vi "Dashboard Main.vi"() -> ()   [LabVIEW 2013]
uses:
  Sally_Framework_2014/AutoEnum.ctl
  Sally_Framework_2014/LauncherPresets.ctl
  Sally_Framework_2014/AutoInstructArray.ctl
  Sally_Framework_2014/AutoInstruction.ctl
  <vilib>/event_ctls.llb/eventvkey.ctl
  DBNameEnum.ctl
  <vilib>/Utility/config.llb/Read Key (String).vi
  <vilib>/Utility/config.llb/Read Key (I32).vi
  <vilib>/Utility/config.llb/Write Key (String).vi
  <vilib>/Utility/config.llb/Write Key (I32).vi
  <vilib>/Utility/config.llb/NI_LVConfig.lvlib
panel:
  out "Battery Value":dbl(slide) scale=0.0..14.0 scale format="%#_2e"
  out "Battery":sgl(graph)
  in  "Camera Settings":T1={"Frate Rate"=30, "Compression"=30, "Size"=1} {"Frate Rate" scale=1.0..30.0; "Size" items=["640x480", "320x240", "160x120"]}
  out "Mode":T2(ring)=enum."Auto Disabled"
  out "Camera IP":string
  out "Robot IP":string
  in  "Dashboard Tab":T3(tab)
  out "ReverseDrive":bool
  in  "Use2DriveAlign":bool=TRUE
  out "DriveAlignLSRight":bool
  out "ClimbLS":bool
  in  "UseLauncherPID":bool=TRUE
  in  "UseAngleEncoder":bool=TRUE
  in  "UseLauncherEncoder":bool=TRUE
  out "LauncherAngleMatches":bool
  out "sDriveDistance":dbl
  out "Drive Loop Timing (ms)":u32
  in  "AutoEnum":T4=enum."BehindPyramid"
  out "LauncherMotorValue":dbl
  out "Version":string
  out "LauncherAngle":cluster{dbl, dbl}(knob) scale=0.0..55.0 scale format="%#2_3g"
  out "DriveAlignLSLeft":bool
  out "LauncherRPM":cluster{dbl, dbl}(knob) scale=0.0..4000.0
  in  "Stress TankDrive":bool
  in  "Stress FP":bool
  in  "NumInstr":dbl
  in  "Disabled":T5=[{"Distance/Angle"=10.0, "Speed"=0.0, "Action"=enum."Wait", "NumFrisbees"=0}]
  in  "BehindPyramid":T5=[{"Distance/Angle"=30.0, "Speed"=2390.0, "Action"=enum."Aim", "NumFrisbees"=0}, {"Distance/Angle"=5.0, "Speed"=0.0, "Action"=enum."Wait", "NumFrisbees"=0}, {"Distance/Angle"=0.0, "Speed"=0.0, "Action"=enum."Shoot", "NumFrisbees"=4}]
  in  "CloseLeft":T5=[{"Distance/Angle"=34.0, "Speed"=2390.0, "Action"=enum."Aim", "NumFrisbees"=0}, {"Distance/Angle"=5.0, "Speed"=0.0, "Action"=enum."Wait", "NumFrisbees"=0}, {"Distance/Angle"=0.0, "Speed"=0.0, "Action"=enum."Shoot", "NumFrisbees"=4}]
  in  "CloseRight":T5=[{"Distance/Angle"=34.0, "Speed"=2390.0, "Action"=enum."Aim", "NumFrisbees"=0}, {"Distance/Angle"=5.0, "Speed"=0.0, "Action"=enum."Wait", "NumFrisbees"=0}, {"Distance/Angle"=0.0, "Speed"=0.0, "Action"=enum."Shoot", "NumFrisbees"=4}]
  in  "BackLeft":T5=[{"Distance/Angle"=29.0, "Speed"=2390.0, "Action"=enum."Aim", "NumFrisbees"=0}, {"Distance/Angle"=5.0, "Speed"=0.0, "Action"=enum."Wait", "NumFrisbees"=0}, {"Distance/Angle"=0.0, "Speed"=0.0, "Action"=enum."Shoot", "NumFrisbees"=4}]
  in  "BackRight":T5=[{"Distance/Angle"=29.0, "Speed"=2390.0, "Action"=enum."Aim", "NumFrisbees"=0}, {"Distance/Angle"=5.0, "Speed"=0.0, "Action"=enum."Wait", "NumFrisbees"=0}, {"Distance/Angle"=0.0, "Speed"=0.0, "Action"=enum."Shoot", "NumFrisbees"=4}]
  in  "BackupAuto":dbl[](array[numeric])=[2390.0, 30.0, 3.0, 4.0, 2000.0, -0.5]
  in  "UseClusterArray":bool
  in  "PullbackTol":dbl=100.0
  in  "FireTol":dbl=10.0
  in  "LauncherRPMTol":dbl=10.0
  in  "LauncherAngleTol":dbl=0.1
  in  "InitialWait (ms)":dbl=5000.0
  in  "WaitBetweenLaunch (ms)":dbl=1200.0
  in  "QSWaitBeforeFire (ms)":dbl=600.0
  in  "QSWaitBeforeRetract (ms)":dbl=100.0
  in  "AngleForwardValue":dbl=0.8
  in  "AngleBackwardValue":dbl=-0.8
  in  "HalfSpeedFactor":dbl=0.75
  in  "RPMPresets":T7={"cPresetPyramid"=2390.0, "cPresetShort"=2390.0, "cPresetMid"=1950.0, "cPresetFar"=2390.0, "cPresetClimbHigh"=0.0, "cPresetClimbLow"=0.0}
  in  "AnglePresets":T7={"cPresetPyramid"=30.0, "cPresetShort"=50.0, "cPresetMid"=51.5, "cPresetFar"=25.0, "cPresetClimbHigh"=32.0, "cPresetClimbLow"=20.0}
  in  "Slider":dbl(slide) scale=0.0..100.0 scale format="%#_3g"
  in  "On/Off":bool caption="Solenoid"
  in  "Test Name":u16(ring) items=["Select the test to run...", "Example Test", "-------------------------------", "List of tests is built in robot code.", "Replace with your own automated tests."]
  in  "Test Tree":string(tree)
  in  "Motor":cluster{"Value":dbl, "Enable":bool} {"Value" scale=-1.0..1.0 scale format="%#_3g"}
  out "Progress":T8 {"Test Progress" scale=0.0..100.0}
  in  "Rev/Fwd":cluster{"Forward":bool, "Reverse":bool}
  in  "Ring":u16(ring) items=["Auto", "Fixed indoor", "Fixed outdoor 1", "Fixed outdoor 2", "Fixed fluorescent 1", "Fixed fluorescent 2", "Hold current"]
  in  "Listbox":i32(listbox)=8
  in  "Viewer":T9(tab)
  out "Mbps":dbl format="%#.1g"
  in  "Enable":bool=TRUE
  in  "DB Camera Config":bool
  out "Mbps":bool
  out "fps":dbl format="%#.1g"
  out "Image Error Message":string="Timeout in Camera Communications"
  out "Camera Image":T10(plugin-control)
  out "Buttons 1":cluster{"1":bool, "2":bool, "3":bool}
  out "Kinect 1":cluster{"X":dbl, "Y":dbl, "Z":dbl} {"X" scale=1.0..-1.0; "Y" scale=1.0..-1.0; "Z" scale=1.0..-1.0}
  out "Buttons 2":cluster{"1":bool, "2":bool, "3":bool}
  out "Kinect 2":cluster{"X":dbl, "Y":dbl, "Z":dbl} {"X" scale=1.0..-1.0; "Y" scale=1.0..-1.0; "Z" scale=1.0..-1.0}
  out "Version":string
  out "Skeleton Picture":picture
  out "Players":i8
  out "Tree":string(tree)
  # "Drive & Motors"
  # "Robot IP:"
  # "sLauncherRPM"
  # "TargetLauncherRPM"
  # "sLauncherAngle"
  # "LauncherTargetAngle"
  # "RPM"
  # "Angle"
  # "Wait (s)"
  # "ShootNum"
  # "Time (ms)"
  # "Motor Value"
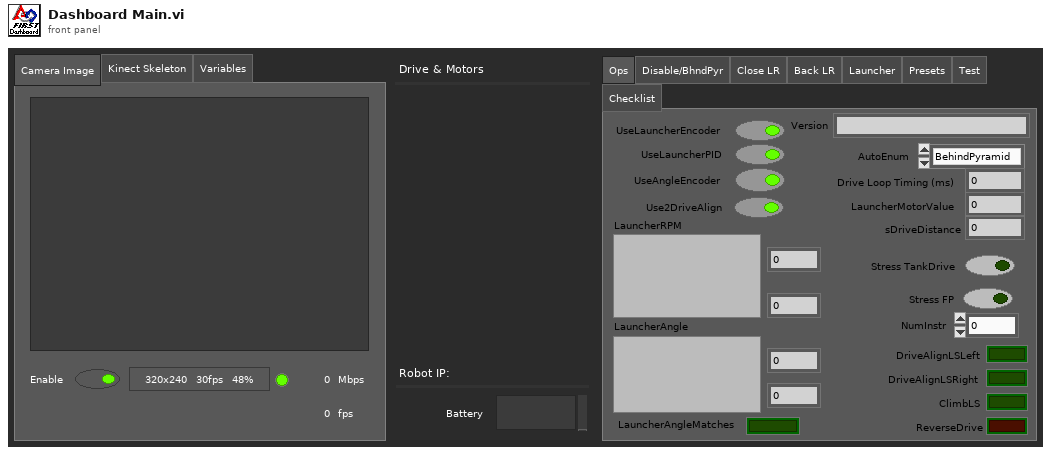
[diagram p1: front panel]
types:
  T1 = cluster{"Frate Rate":i32, "Compression":i32, "Size":u16}
  T2 = enum8{"Tele-Op Disabled", "Tele-Op Enabled", "Auto Disabled", "Auto Enabled", "Test Disabled", "Test Enabled", ""}
  T3 = enum32{"Ops", "Disable/BhndPyr", "Close LR", "Back LR", "Launcher", "Presets", "Test", "Checklist"}
  T4 = typedef "AutoEnum.ctl" = enum16{"Disabled", "BackRight", "BackLeft", "CloseRight", "CloseLeft", "BehindPyramid"}
  T5 = typedef "AutoInstructArray.ctl" = T6[]
  T6 = typedef "AutoInstruction.ctl" = cluster{"Distance/Angle":dbl, "Speed":dbl, "Action":enum16{"DriveForward", "Turn", "Aim", "Shoot", "Wait"}, "NumFrisbees":i32}
  T7 = typedef "LauncherPresets.ctl" = cluster{"cPresetPyramid":dbl, "cPresetShort":dbl, "cPresetMid":dbl, "cPresetFar":dbl, "cPresetClimbHigh":dbl, "cPresetClimbLow":dbl}
  T8 = cluster{"Test Progress":u8, "Test Progress Text":string}
  T9 = enum32{"Camera Image", "Kinect Skeleton", "Variables"}
  T10 = typedef "IMAQ Image.ctl" = refnum<image>
  T11 = typedef "Image Type" = u32
  T12 = typedef "LVBoundsTypeDef.ctl" = cluster{"Width":u32, "Height":u32}
  T13 = typedef "SkeletonTrackState.ctl" = enum32{"NotTracked", "PositionOnly", "Tracked"}
  T14 = cluster{"TrackingState":u8[], "Position":cluster{"x":sgl, "y":sgl, "z":sgl}, cluster{"x":sgl, "y":sgl, "z":sgl, sgl}[], "TrackState":T13}
  T15 = cluster{cluster{"ScaledToPercentRange":dbl, "ScaledToPercentRange":dbl, "ScaledToPercentRange":dbl}, cluster{bool, bool, bool}}[]
  T16 = cluster{cluster{"ScaledToPercentRange":dbl, "ScaledToPercentRange":dbl, "ScaledToPercentRange":dbl}, cluster{bool, bool, bool}}
  T17 = cluster{"ScaledToPercentRange":dbl, "ScaledToPercentRange":dbl, "ScaledToPercentRange":dbl}
  T18 = typedef "LVRectTypeDef.ctl" = cluster{"Left":i16, "Top":i16, "Right":i16, "Bottom":i16}
  T19 = typedef "DBNameEnum.ctl" = enum16{"AutoInstructions", "DriveLoopTime", "DriveAlignLSLeft", "DriveAlignLSRight", "Use2DriveAlign", "ClimbLS", "LauncherAngleMatches", "FrameworkVersion", "sLauncherAngle", "LauncherTargetAngle", "sLauncherRPM", "LauncherTargetRPM", "sDriveDistance", "LauncherMotorValue", "PullbackTol", "FireTol", "LauncherRPMTol", "LauncherAngleTol", "InitialWait", "WaitBetweenLaunch", "AnglePresets", "RPMPresets", "UseAngleEncoder", "UseLauncherEncoder", "UseLauncherPID", "QSWaitBeforeFire", "QSWaitBeforeRetract", "AngleForwardValue", "AngleBackwardValue", "UseClusterArray", "BackupAuto", "ReverseDriveIndicate", "HalfSpeedFactor"}
  T20 = cluster{"Competition mode":bool, "Robot Link":bool, "Autonomous":bool, "Enabled":bool, "E-Stop":bool, "Simulated":bool, "TestMode":bool, "Docked Window":bool}
  T21 = typedef "NI_LVConfig.lvlib/Config Data RefNum.ctl" = refnum<k1>
  T22 = typedef "eventvkey.ctl" = enum16{"ASCII", "Enter", "Return", "Shift", "Ctrl", "Alt", "Cmd", "Opt", "Caps", "NumLock", "Clear", "Break", "Up", "Down", "Left", "Right", "Insert", "Delete", "Home", "End", "PageUp", "PageDown", "Escape", "Help", "Pause", "ScrollLock", "F1", "F2", "F3", "F4", "F5", "F6", "F7", "F8", "F9", "F10", "F11", "F12", "F13", "F14", "F15", "F16", "F17", "F18", "F19", "F20", "F21", "F22", "F23", "F24", "Play", "VolumeUp", "VolumeDown", "Mute", "Two Byte Char"}
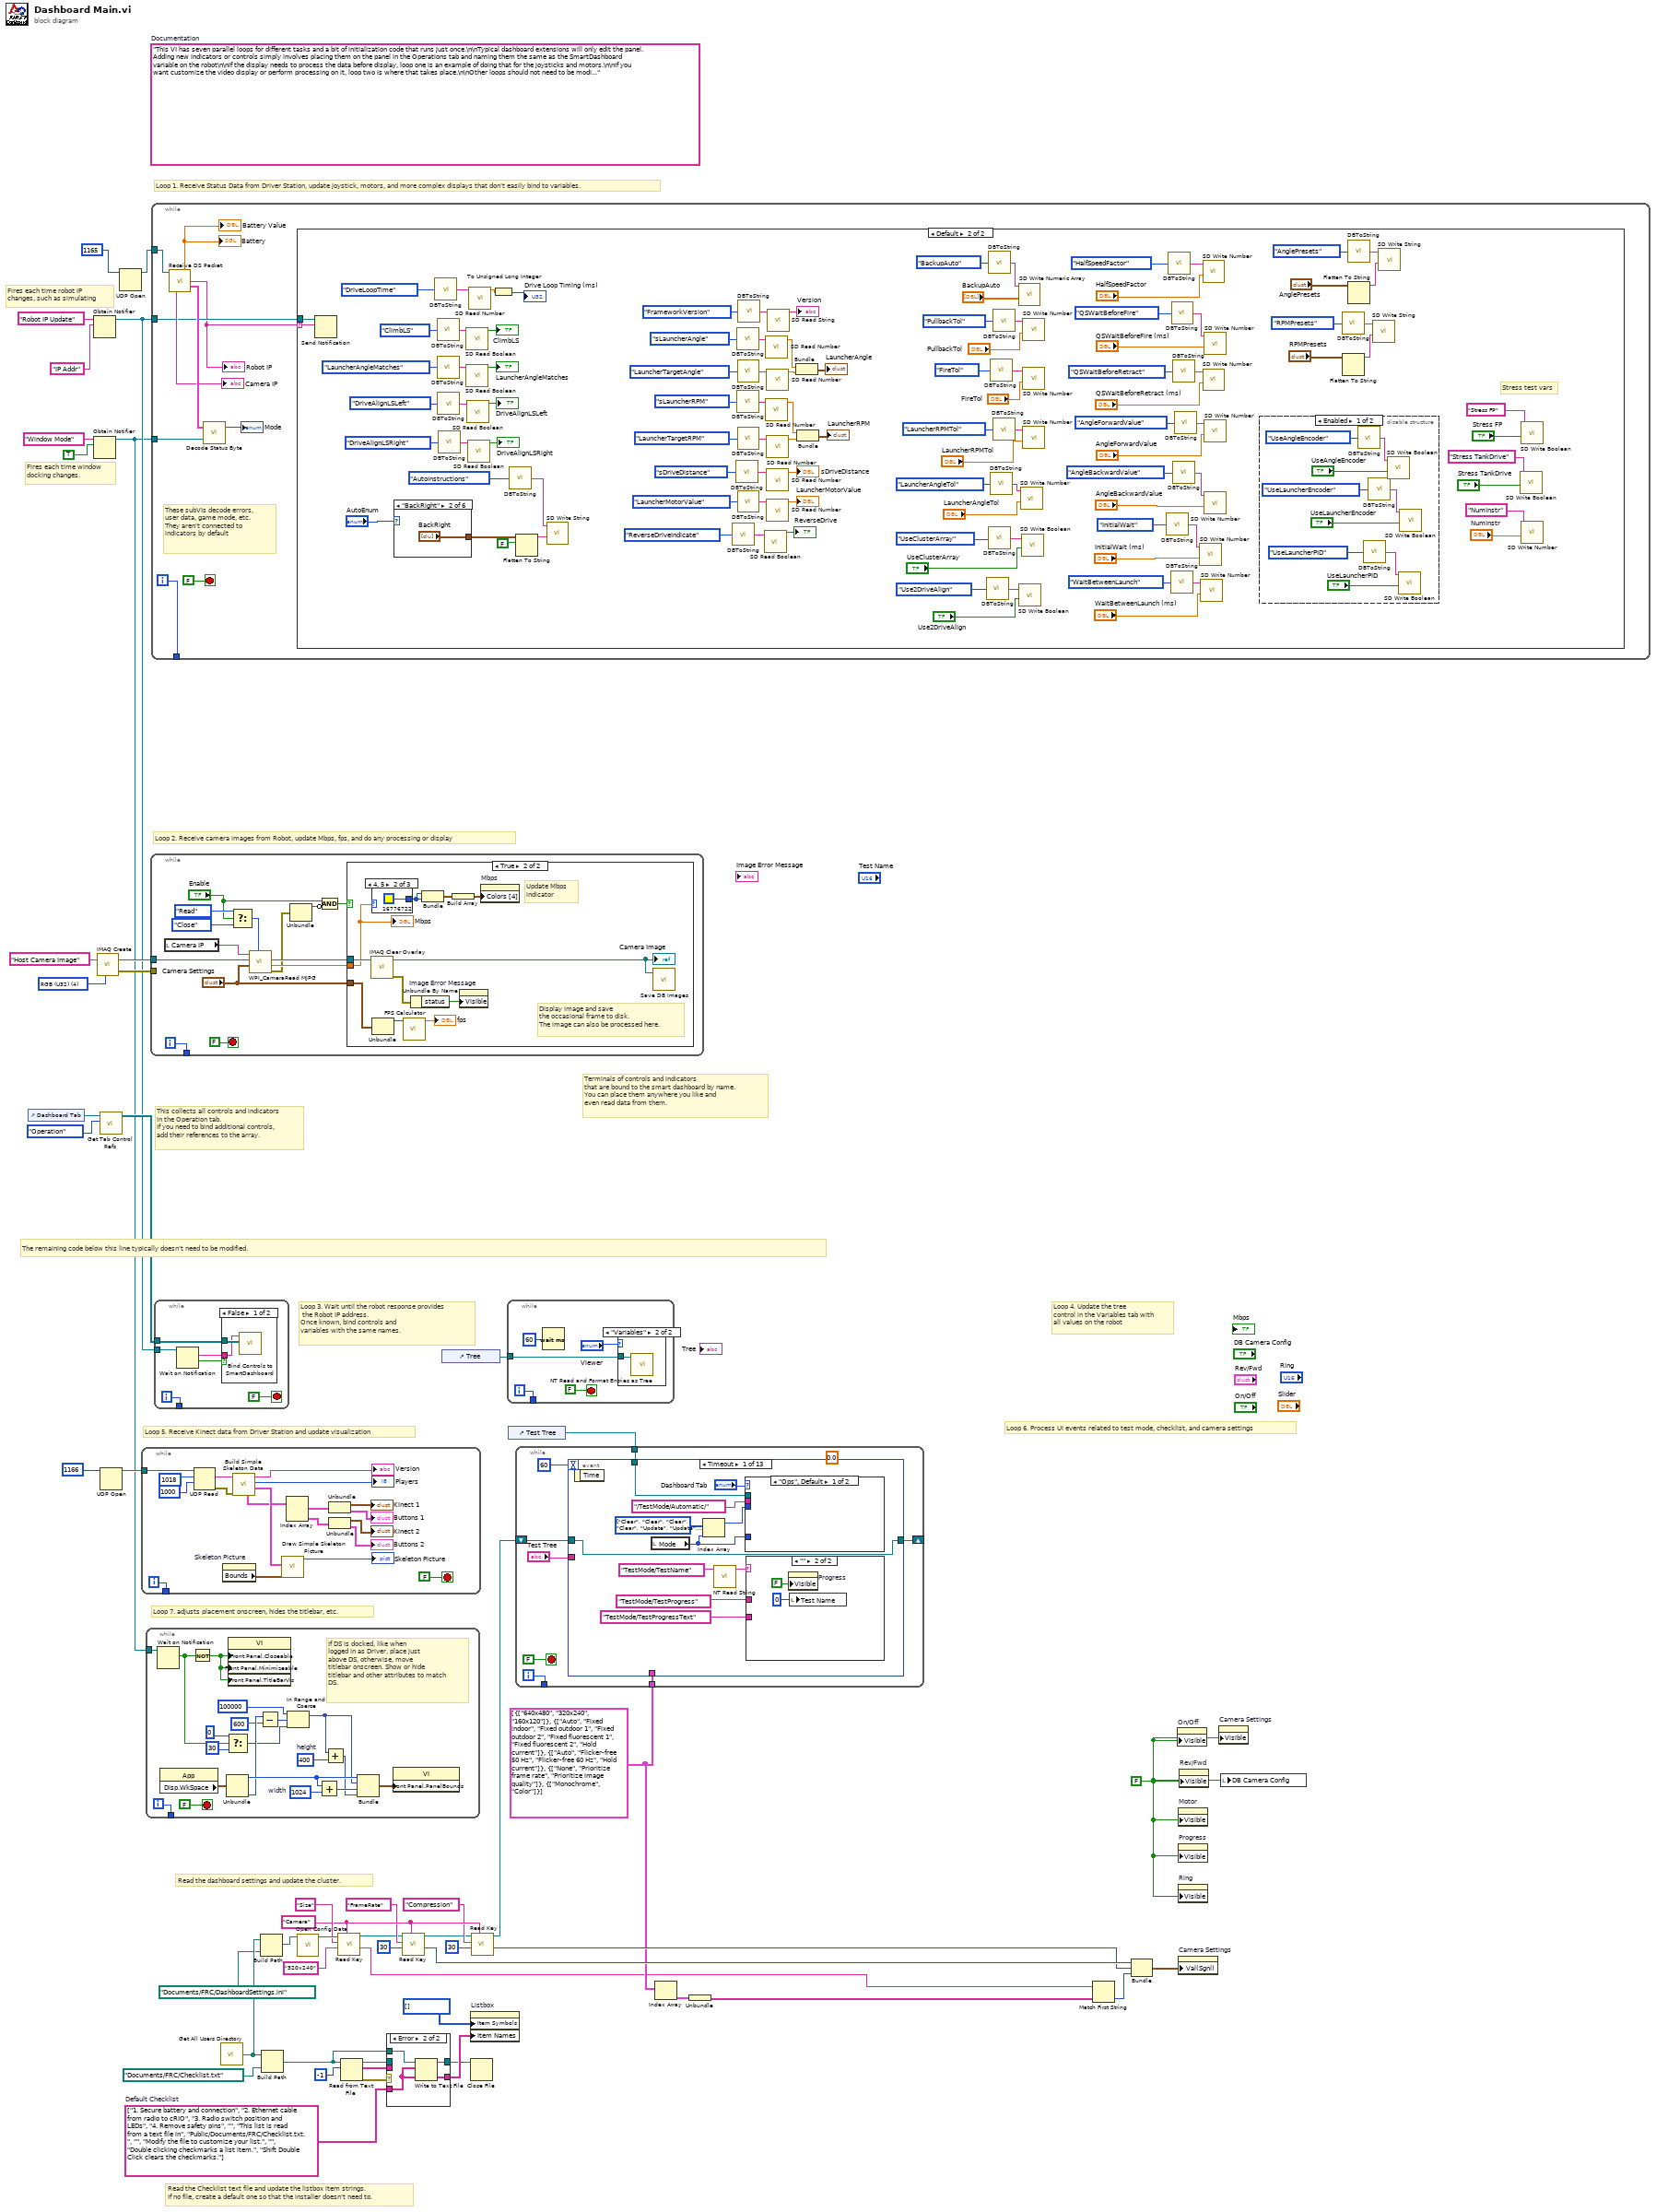
[diagram p0: block diagram]
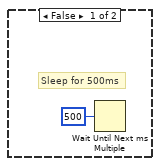
[diagram p3: hidden frame]
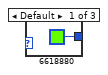
[diagram p4: hidden frame]
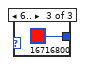
[diagram p5: hidden frame]
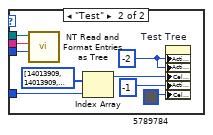
[diagram p7: hidden frame]
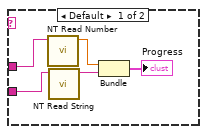
[diagram p8: hidden frame]
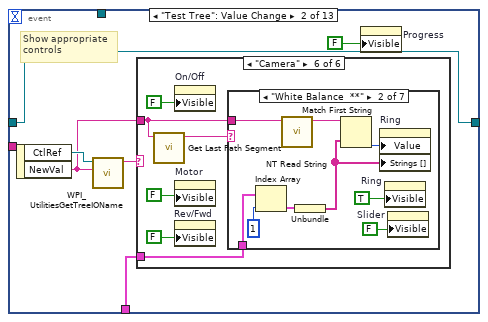
[diagram p9: hidden frame]
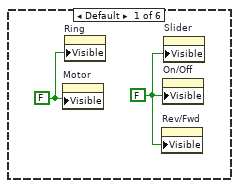
[diagram p10: hidden frame]
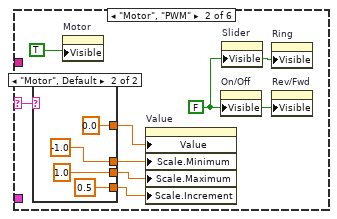
[diagram p11: hidden frame]
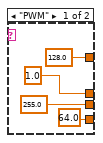
[diagram p12: hidden frame]
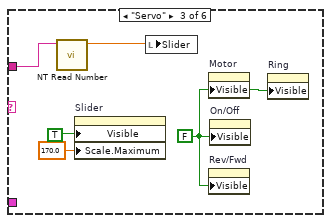
[diagram p13: hidden frame]
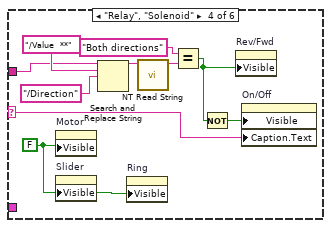
[diagram p14: hidden frame]
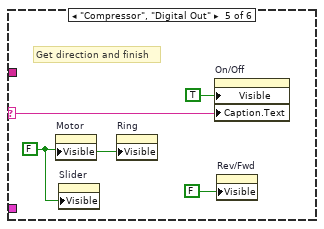
[diagram p15: hidden frame]
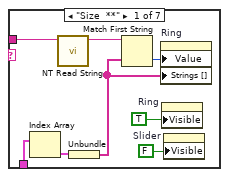
[diagram p16: hidden frame]
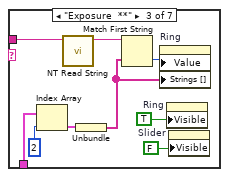
[diagram p17: hidden frame]
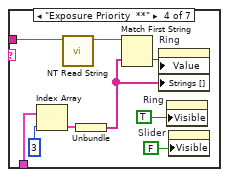
[diagram p18: hidden frame]
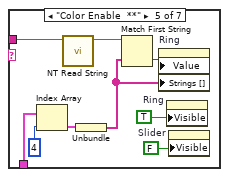
[diagram p19: hidden frame]
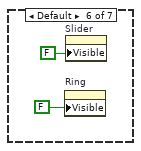
[diagram p20: hidden frame]
diagram:
  w21 = "Camera"
  w13 = cluster{string[]}[] [{["640x480", "320x240", "160x120"]}, {["Auto", "Fixed indoor", "Fixed outdoor 1", "Fixed outdoor 2", "Fixed fluorescent 1", "Fixed fluorescent 2", "Hold current"]}, {["Auto", "Flicker-free 50 Hz", "Flicker-free 60 Hz", "Hold current"]}, {["None", "Prioritize frame rate", "Prioritize image quality"]}, {["Monochrome", "Color"]}]
  w29 = string[] ["1. Secure battery and connection", "2. Ethernet cable from radio to cRIO", "3. Radio switch position and LEDs", "4. Remove safety pins", "", "This list is read from a text file in", "Public/Documents/FRC/Checklist.txt.", "", "Modify the file to customize your list.", "", "Double clicking checkmarks a list item.", "Shift Double Click clears the checkmarks."]  # Default Checklist
  w27 = FALSE ("Visible")
  (unwired) "This VI has seven parallel loops for different tasks and a bit of initialization code that runs just once.\n\nTypical dashboard extensions will only edit the panel. Adding new indicators or controls simply involves placing them on the panel in the Operations tab and naming them the same as the SmartDashboard variable on the robot\n\nIf the display needs to process the data before display, loop one is an example of doing that for the joysticks and motors.\n\nIf you want customize the video display or perform processing on it, loop two is where that takes place.\n\nOther loops should not need to be modified. They are pretty standard, and document the task they perform."  # Documentation
  w50 = T11 4 items=["Grayscale (U8)", "Grayscale (I16)", "Grayscale (SGL)", "Complex (CSG)", "RGB (U32)", "HSL (U32)", "RGB (U64)"] ("Image Type")
  # "Fires each time robot IP\nchanges, such as simulating"
  # "Fires each time window\ndocking changes."
  # "Read the Checklist text file and update the listbox item strings.\nIf no file, create a default one so that the installer doesn't need to."
  # "This collects all controls and indicators\nin the Operation tab.\nIf you need to bind additional controls,\nadd their references to the array."
  # "The remaining code below this line typically doesn't need to be modified."
  # "Loop 6. Process UI events related to test mode, checklist, and camera settings"
  # "Read the dashboard settings and update the cluster."
  # "Terminals of controls and indicators\nthat are bound to the smart dashboard by name.\nYou can place them anywhere you like and\neven read data from them."
  # "Loop 4. Update the tree\ncontrol in the Variables tab with\nall values on the robot"
  # "Loop 3. Wait until the robot response provides\n the Robot IP address.\nOnce known, bind controls and\nvariables with the same names."
  # "Loop 5. Receive Kinect data from Driver Station and update visualization"
  # "Loop 7. adjusts placement onscreen, hides the titlebar, etc."
  # "Loop 1. Receive Status Data from Driver Station, update joystick, motors, and more complex displays that don't easily bind to variables."
  # "Loop 2. Receive camera images from Robot, update Mbps, fps, and do any processing or display"
  n1 = control-ref of="Dashboard Tab"() -> (w43:refnum<vi>)
  n2 = Obtain Notifier(name (unnamed)="Robot IP Update", notification data type="IP Addr" ("name (unnamed)")) -> (notifier out=w40:refnum<notifier>)  [unwired: 2 in, 2 out]
  n3 = Obtain Notifier(name (unnamed)="Window Mode", notification data type=TRUE) -> (notifier out=w33:refnum<notifier>)  [unwired: 2 in, 2 out]
  n4 = call "IMAQ Create"("Image Name"="Host Camera Image", "Image Type"=w50) -> ("New Image"=w48:T10, "error out"=w47:errorcluster)  [unwired: 2 in, 1 out]
  n5 = call <vilib>:"Get Tab Control Refs.vi"("Page Index"=enum32{"Operation", "Test"}."Operation" ("Dashboard Tab"), "TabControl in"=w43) -> ("ControlsOnPage"=w44:refnum<vi>[])  [unwired: 9 in]
  n6 = UDP Open(11:u16 1166 ("port")) -> (port=w45:refnum<k16>)  [unwired: 2 in, 4 out]
  n7 = UDP Open(11:u16 1165 ("port")) -> (port=w51:refnum<k16>)  [unwired: 2 in, 4 out]
  n8 = while {
    tunnel: w45 -> [w69]
    tunnel: [w54] -> _
    i -> [w54]
    stop <- FALSE stop-if-true
    n9 = UDP Read(connection ID=w69, max size (548)=1018 ("bytes to read"), timeout ms (25000)=1000) -> (data out=w63:string, error out=w53:errorcluster)  [unwired: 1 in, 3 out]
    n10 = property on="Skeleton Picture" class="Pict"() -> ("Bounds"=w65:T12)  [unwired: 2 in, 2 out]
    n11 = call "Build Simple Skeleton Data.vi"("error in (no error)"=w53, "data in"=w63) -> ("Skeleton Data"=w64:T14, "NumPlayers"=→"Players":i8, "Version String"=→"Version":string, "Simple Joystick Info"=w61:T15)  [unwired: 5 in, 1 out]
    n12 = call "Draw Simple Skeleton Picture.vi"("Bounds"=w65, "Simple Skeleton"=w64) -> ("new picture out"=→"Skeleton Picture":picture)  [unwired: 9 in]
    n13 = Index Array(array=w61) -> (element #1=w60:T16, element #2=w59:T16)  [unwired: 2 in]
    n14 = Unbundle(w60) -> (→"Kinect 1":T17, →"Buttons 1":cluster{bool, bool, bool})
    n15 = Unbundle(w59) -> (→"Kinect 2":T17, →"Buttons 2":cluster{bool, bool, bool})
  }
  n16 = while {
    tunnel: w33 -> [w90]
    tunnel: [w88] -> _
    i -> [w88]
    stop <- FALSE stop-if-true
    w80 = 1024  # width
    w83 = 400  # height
    # "If DS is docked, like when\nlogged in as Driver, place just\nabove DS, otherwise, move\ntitlebar onscreen. Show or hide\ntitlebar and other attributes to match\nDS."
    n17 = Wait on Notification(notifier=w90) -> (notification=w75:bool)  [unwired: 3 in, 3 out]
    n18 = property class="App"() -> ("Disp.WkSpace"=w86:T18)  [unwired: 2 in, 2 out]
    n19 = Not(x=w75) -> (.not. x?=w89:bool)
    n20 = Unbundle(w86) -> ("Left"=w84:i16, "Bottom"=w81:i16)  [unwired: 2 out]
    n21 = Select(t=0, s=w75, f=30) -> (s? t:f=w74:i32)
    n22 = property class="VI"("Front Panel.Closeable"=w89, "Front Panel.Minimizeable"=w89, "Front Panel.TitleBarVis"=w89) -> ()  [unwired: 2 in, 2 out]
    n23 = Subtract(x=w81, y=600) -> (x-y=w78:i32)
    n24 = In Range and Coerce(upper limit=100000, x=w78, lower limit=w74) -> (coerced(x)=w72:i32)  [unwired: 1 out]
    n25 = Add(x=w84, y=w80) -> (x+y=w85:i32)
    n26 = Add(x=w72, y=w83) -> (x+y=w82:i32)
    n27 = Bundle("Left"=w84, w72, w85, w82) -> (w87:cluster{"Left":i16, i32, i32, i32})  [unwired: 1 out]
    n28 = property class="VI"("Front Panel.PanelBounds"=w87) -> ()  [unwired: 2 in, 2 out]
  }
  n29 = while {
    tunnel: w48 -> [w101]
    tunnel: w47 -> [_]
    tunnel: [w104] -> _
    i -> [w104]
    stop <- FALSE stop-if-true
    n30 = local read "Camera IP"() -> (w103:string)
    n31 = Select(t=enum16{"Read", "Reopen", "Close"}."Read" ("Operation"), s="Enable", f=enum16{"Read", "Reopen", "Close"}."Close" ("Operation")) -> (s? t:f=w96:enum16{"Read", "Reopen", "Close"})
    n32 = call <vilib>:"WPI_CameraRead MJPG.vi"("Operation"=w96, "Camera Settings"="Camera Settings", "Image"=w101, "address"=w103) -> ("error out"=w95:errorcluster, "Bandwidth (Mbps)"=w99:dbl, "Image Out"=w100:T10)  [unwired: 5 in]
    n33 = Unbundle(w95) -> ("status"=w93:bool)  [unwired: 2 out]
    n34 = Compound Arithmetic op=AND("Enable", invert w93) -> (w92:bool)
    n35 = case shown="True" w92 {
      tunnel: "Camera Settings" -> [_ w108]
      tunnel: w100 -> [_ w111]
      tunnel: w99 -> [_ w110]
      frame False {
        # "Sleep for 500ms"
        n36 = Wait Until Next ms Multiple(millisecond multiple=u32 500) -> ()  [unwired: 1 out]
      }
      frame True {
        # "Display image and save\nthe occasional frame to disk.\nThe image can also be processed here."
        # "Update Mbps\nindicator"
        n37 = call "IMAQ Clear Overlay"("Image"=w111) -> ("error out"=w116:errorcluster, "Image Out"=w115:T10)  [unwired: 2 in, 7 out]
        "Camera Image" <- w115
        n38 = case shown="4, 5" w110 {
          tunnel: [u32 6618880 ("Color Box") u32 16776722 ("Color Box") u32 16716800 ("Color Box")] -> w112
          frame Default {
          }
          frame 4, 5 {
          }
          frame 6.. {
          }
        }
        n39 = Unbundle(w108) -> ("Frate Rate"=w107:i32)  [unwired: 2 out]
        n40 = call "FPS Calculator.vi"("Average Count"=w107) -> ("fps"=→"fps":dbl)  [unwired: 10 in]
        n41 = Unbundle By Name(w116) -> ("status"=w117:bool)
        n42 = Bundle("Color Box"=w112, "Color Box"=w112) -> (w114:cluster{"Color Box":u32, "Color Box":u32})  [unwired: 1 out]
        n43 = Build Array(w114) -> (w113:cluster{"Color Box":u32, "Color Box":u32}[])
        n44 = property on="Image Error Message" class="Str"("Visible"=w117) -> ()  [unwired: 2 in, 2 out]
        n45 = property on="Mbps" class="Bool (strict)"("Colors [4]"=w113) -> ()  [unwired: 2 in, 2 out]
        n46 = call "Save DB Images.vi"("Image"=w115) -> ()  [unwired: 2 in, 1 out]
        "Mbps" <- w110
      }
    }
  }
  n47 = while {
    tunnel: w51 -> [w128]
    tunnel: w40 -> [w122]
    tunnel: w33 -> [w126]
    tunnel: [w123] -> _
    i -> [w123]
    stop <- FALSE stop-if-true
    # "These subVIs decode errors, user data, game mode, etc.\nThey aren't connected to indicators by default"
    n48 = call "Receive DS Packet.vi"("Recv Socket"=w128) -> ("Battery"=→"Battery" →"Battery Value":sgl, "Robot IP Address"=w121:string, "Status"=w129:T20, "Camera IP Address"=→"Camera IP":string)  [unwired: 1 in, 10 out]
    "Robot IP" <- w121
    n49 = call "Decode Status Byte.vi"("Window Mode Notifier"=w126, "Status"=w129) -> ("Mode"=→"Mode":T2)  [unwired: 1 out]
    n50 = case shown="Default" w121 {
      selector: w121 -> [_ w235]
      tunnel: w122 -> [_ w236]
      frame "0.0.0.0" {
        # "Robot not responding, don't poll the variables"
      }
      frame Default {
        # "Stress test vars"
        n51 = Send Notification(notification=w235, notifier=w236) -> ()  [unwired: 1 in, 2 out]
        n52 = case shown="\"BackRight\"" "AutoEnum" {
          tunnel: ["Disabled" "BackRight" "BackLeft" "CloseRight" "CloseLeft" "BehindPyramid"] -> w170
          frame "Disabled" {
          }
          frame "BackRight" {
          }
          frame "BackLeft" {
          }
          frame "CloseRight" {
          }
          frame "CloseLeft" {
          }
          frame "BehindPyramid", Default {
          }
        }
        n53 = call "DBToString.vi"("Enum"=DBNameEnum."DriveLoopTime") -> ("Refname"=w168:string)
        n54 = call "DBToString.vi"("Enum"=DBNameEnum."ClimbLS") -> ("Refname"=w176:string)
        n55 = call "DBToString.vi"("Enum"=DBNameEnum."LauncherAngleMatches") -> ("Refname"=w175:string)
        n56 = call "DBToString.vi"("Enum"=DBNameEnum."DriveAlignLSLeft") -> ("Refname"=w179:string)
        n57 = call "DBToString.vi"("Enum"=DBNameEnum."DriveAlignLSRight") -> ("Refname"=w167:string)
        n58 = call <vilib>:"SD Read Boolean.vi"("Name"=w176) -> ("Boolean"=→"ClimbLS":bool)  [unwired: 8 in, 2 out]
        n59 = call <vilib>:"SD Read Boolean.vi"("Name"=w175) -> ("Boolean"=→"LauncherAngleMatches":bool)  [unwired: 8 in, 2 out]
        n60 = call <vilib>:"SD Read Boolean.vi"("Name"=w179) -> ("Boolean"=→"DriveAlignLSLeft":bool)  [unwired: 8 in, 2 out]
        n61 = call <vilib>:"SD Read Boolean.vi"("Name"=w167) -> ("Boolean"=→"DriveAlignLSRight":bool)  [unwired: 8 in, 2 out]
        n62 = call <vilib>:"SD Read Number.vi"("Name"=w168) -> ("Numeric"=w234:dbl)  [unwired: 8 in, 2 out]
        n63 = To Unsigned Long Integer(number=w234) -> (unsigned 32bit integer=→"Drive Loop Timing (ms)":u32)
        n64 = call "DBToString.vi"("Enum"=DBNameEnum."AutoInstructions") -> ("Refname"=w173:string)
        n65 = Flatten To String(anything=w170, prepend array or string size? (T)=FALSE) -> (data string=w171:string)  [unwired: 2 in, 2 out]
        n66 = call <vilib>:"SD Write String.vi"("String"=w171, "Name"=w173) -> ()  [unwired: 8 in, 2 out]
        n67 = call "DBToString.vi"("Enum"=DBNameEnum."ReverseDriveIndicate") -> ("Refname"=w140:string)
        n68 = call "DBToString.vi"("Enum"=DBNameEnum."sDriveDistance") -> ("Refname"=w181:string)
        n69 = call "DBToString.vi"("Enum"=DBNameEnum."sLauncherAngle") -> ("Refname"=w187:string)
        n70 = call "DBToString.vi"("Enum"=DBNameEnum."sLauncherRPM") -> ("Refname"=w185:string)
        n71 = call "DBToString.vi"("Enum"=DBNameEnum."LauncherTargetAngle") -> ("Refname"=w186:string)
        n72 = call "DBToString.vi"("Enum"=DBNameEnum."LauncherTargetRPM") -> ("Refname"=w184:string)
        n73 = call "DBToString.vi"("Enum"=DBNameEnum."LauncherMotorValue") -> ("Refname"=w193:string)
        n74 = call "DBToString.vi"("Enum"=DBNameEnum."FrameworkVersion") -> ("Refname"=w183:string)
        n75 = call <vilib>:"SD Read Boolean.vi"("Name"=w140) -> ("Boolean"=→"ReverseDrive":bool)  [unwired: 8 in, 2 out]
        n76 = call <vilib>:"SD Read Number.vi"("Name"=w187) -> ("Numeric"=w220:dbl)  [unwired: 8 in, 2 out]
        n77 = call <vilib>:"SD Read Number.vi"("Name"=w185) -> ("Numeric"=w216:dbl)  [unwired: 8 in, 2 out]
        n78 = call <vilib>:"SD Read Number.vi"("Name"=w186) -> ("Numeric"=w221:dbl)  [unwired: 8 in, 2 out]
        n79 = call <vilib>:"SD Read Number.vi"("Name"=w184) -> ("Numeric"=w217:dbl)  [unwired: 8 in, 2 out]
        n80 = call <vilib>:"SD Read Number.vi"("Name"=w181) -> ("Numeric"=→"sDriveDistance":dbl)  [unwired: 8 in, 2 out]
        n81 = call <vilib>:"SD Read Number.vi"("Name"=w193) -> ("Numeric"=→"LauncherMotorValue":dbl)  [unwired: 8 in, 2 out]
        n82 = call <vilib>:"SD Read String.vi"("Name"=w183) -> ("String"=→"Version":string)  [unwired: 8 in, 2 out]
        n83 = Bundle("Numeric"=w220, "Numeric"=w221) -> (→"LauncherAngle":cluster{"Numeric":dbl, "Numeric":dbl})  [unwired: 1 in]
        n84 = Bundle("Numeric"=w216, "Numeric"=w217) -> (→"LauncherRPM":cluster{"Numeric":dbl, "Numeric":dbl})  [unwired: 1 in]
        n85 = call "DBToString.vi"("Enum"=DBNameEnum."Use2DriveAlign") -> ("Refname"=w163:string)
        n86 = call "DBToString.vi"("Enum"=DBNameEnum."BackupAuto") -> ("Refname"=w145:string)
        n87 = call "DBToString.vi"("Enum"=DBNameEnum."UseClusterArray") -> ("Refname"=w148:string)
        n88 = call "DBToString.vi"("Enum"=DBNameEnum."FireTol") -> ("Refname"=w195:string)
        n89 = call "DBToString.vi"("Enum"=DBNameEnum."LauncherAngleTol") -> ("Refname"=w197:string)
        n90 = call "DBToString.vi"("Enum"=DBNameEnum."PullbackTol") -> ("Refname"=w194:string)
        n91 = call "DBToString.vi"("Enum"=DBNameEnum."LauncherRPMTol") -> ("Refname"=w196:string)
        n92 = call <vilib>:"SD Write Numeric Array.vi"("Numeric Array"="BackupAuto", "Name"=w145) -> ()  [unwired: 8 in, 2 out]
        n93 = call <vilib>:"SD Write Boolean.vi"("Boolean"="Use2DriveAlign", "Name"=w163) -> ()  [unwired: 8 in, 2 out]
        n94 = call <vilib>:"SD Write Number.vi"("Numeric"="LauncherAngleTol", "Name"=w197) -> ()  [unwired: 8 in, 2 out]
        n95 = call <vilib>:"SD Write Boolean.vi"("Boolean"="UseClusterArray", "Name"=w148) -> ()  [unwired: 8 in, 2 out]
        n96 = call <vilib>:"SD Write Number.vi"("Numeric"="PullbackTol", "Name"=w194) -> ()  [unwired: 8 in, 2 out]
        n97 = call <vilib>:"SD Write Number.vi"("Numeric"="FireTol", "Name"=w195) -> ()  [unwired: 8 in, 2 out]
        n98 = call <vilib>:"SD Write Number.vi"("Numeric"="LauncherRPMTol", "Name"=w196) -> ()  [unwired: 8 in, 2 out]
        n99 = call "DBToString.vi"("Enum"=DBNameEnum."InitialWait") -> ("Refname"=w209:string)
        n100 = call "DBToString.vi"("Enum"=DBNameEnum."HalfSpeedFactor") -> ("Refname"=w137:string)
        n101 = call "DBToString.vi"("Enum"=DBNameEnum."WaitBetweenLaunch") -> ("Refname"=w208:string)
        n102 = call "DBToString.vi"("Enum"=DBNameEnum."QSWaitBeforeFire") -> ("Refname"=w159:string)
        n103 = call "DBToString.vi"("Enum"=DBNameEnum."QSWaitBeforeRetract") -> ("Refname"=w156:string)
        n104 = call "DBToString.vi"("Enum"=DBNameEnum."AngleBackwardValue") -> ("Refname"=w150:string)
        n105 = call "DBToString.vi"("Enum"=DBNameEnum."AngleForwardValue") -> ("Refname"=w153:string)
        n106 = call <vilib>:"SD Write Number.vi"("Numeric"="InitialWait (ms)", "Name"=w209) -> ()  [unwired: 8 in, 2 out]
        n107 = call <vilib>:"SD Write Number.vi"("Numeric"="WaitBetweenLaunch (ms)", "Name"=w208) -> ()  [unwired: 8 in, 2 out]
        n108 = call <vilib>:"SD Write Number.vi"("Numeric"="HalfSpeedFactor", "Name"=w137) -> ()  [unwired: 8 in, 2 out]
        n109 = call <vilib>:"SD Write Number.vi"("Numeric"="QSWaitBeforeRetract (ms)", "Name"=w156) -> ()  [unwired: 8 in, 2 out]
        n110 = call <vilib>:"SD Write Number.vi"("Numeric"="QSWaitBeforeFire (ms)", "Name"=w159) -> ()  [unwired: 8 in, 2 out]
        n111 = call <vilib>:"SD Write Number.vi"("Numeric"="AngleForwardValue", "Name"=w153) -> ()  [unwired: 8 in, 2 out]
        n112 = call <vilib>:"SD Write Number.vi"("Numeric"="AngleBackwardValue", "Name"=w150) -> ()  [unwired: 8 in, 2 out]
        n113 = disable-structure shown="Enabled" {
          frame Enabled {
            n114 = call "DBToString.vi"("Enum"=DBNameEnum."UseAngleEncoder") -> ("Refname"=w248:string)
            n115 = call "DBToString.vi"("Enum"=DBNameEnum."UseLauncherPID") -> ("Refname"=w243:string)
            n116 = call "DBToString.vi"("Enum"=DBNameEnum."UseLauncherEncoder") -> ("Refname"=w244:string)
            n117 = call <vilib>:"SD Write Boolean.vi"("Boolean"="UseAngleEncoder", "Name"=w248) -> ()  [unwired: 8 in, 2 out]
            n118 = call <vilib>:"SD Write Boolean.vi"("Boolean"="UseLauncherPID", "Name"=w243) -> ()  [unwired: 8 in, 2 out]
            n119 = call <vilib>:"SD Write Boolean.vi"("Boolean"="UseLauncherEncoder", "Name"=w244) -> ()  [unwired: 8 in, 2 out]
          }
          frame Disabled {
          }
        }
        n120 = call "DBToString.vi"("Enum"=DBNameEnum."RPMPresets") -> ("Refname"=w204:string)
        n121 = Flatten To String(anything="RPMPresets") -> (data string=w228:string)  [unwired: 3 in, 2 out]
        n122 = call "DBToString.vi"("Enum"=DBNameEnum."AnglePresets") -> ("Refname"=w203:string)
        n123 = Flatten To String(anything="AnglePresets") -> (data string=w229:string)  [unwired: 3 in, 2 out]
        n124 = call <vilib>:"SD Write String.vi"("String"=w228, "Name"=w204) -> ()  [unwired: 8 in, 2 out]
        n125 = call <vilib>:"SD Write String.vi"("String"=w229, "Name"=w203) -> ()  [unwired: 8 in, 2 out]
        n126 = call <vilib>:"SD Write Boolean.vi"("Boolean"="Stress TankDrive", "Name"="Stress TankDrive") -> ()  [unwired: 8 in, 2 out]
        n127 = call <vilib>:"SD Write Number.vi"("Numeric"="NumInstr", "Name"="NumInstr") -> ()  [unwired: 8 in, 2 out]
        n128 = call <vilib>:"SD Write Boolean.vi"("Boolean"="Stress FP", "Name"="Stress FP") -> ()  [unwired: 8 in, 2 out]
      }
    }
  }
  n129 = while {
    tunnel: w44 -> [w257]
    tunnel: w40 -> [w254]
    tunnel: [w252] -> _
    i -> [w252]
    stop <- FALSE stop-if-true
    n130 = Wait on Notification(notifier=w254) -> (notification=w253:string, timed out?=w255:bool)  [unwired: 3 in, 2 out]
    n131 = case shown="False" w255 {
      tunnel: w257 -> [w259 _]
      tunnel: w253 -> [w258 _]
      frame False {
        n132 = call <vilib>:"Bind Controls to SmartDashboard.vi"("Bound Control Refs"=w259, "Server IP Address"=w258) -> ()  [unwired: 10 in]
      }
      frame True {
      }
    }
  }
  n133 = call "Get All Users Directory.vi"() -> ("All User Path"=w26:path)
  n134 = Build Path(base path=w26, name or relative path=path "Documents/FRC/DashboardSettings.ini") -> (appended path=w25:path)
  n135 = Build Path(base path=w26, name or relative path=path "Documents/FRC/Checklist.txt") -> (appended path=w30:path)
  n136 = call <vilib>:"Open Config Data.vi"("configuration file path"=w25) -> ("refnum"=w24:T21)  [unwired: 8 in, 2 out]
  n137 = call-poly <vilib>:"Read Key.vi"("section"=w21, "default value"="320x240", "key"="Size", "refnum"=w24) -> ("value"=w11:string, "refnum out"=w6:T21)  [unwired: 2 in, 4 out]
  n138 = Read from Text File(file (use dialog)=w30, count=-1 ("timeout ms (25000)")) -> (refnum out=w8:refnum<file>, text=w31:string[], error out=w32:errorcluster)  [unwired: 2 in, 1 out]
  n139 = case shown="Error" w32 {
    tunnel: w31 -> [w261 _]
    tunnel: [w261 w263] -> w28
    tunnel: w29 -> [_ w263]
    tunnel: w30 -> [_ w264]
    tunnel: [w260 w262] -> w7
    tunnel: w8 -> [w260 _]
    frame No Error {
    }
    frame Error {
      n140 = Write to Text File(file (use dialog)=w264, text=w263) -> (refnum out=w262:refnum<file>)  [unwired: 2 in, 2 out]
    }
  }
  n141 = call-poly <vilib>:"Read Key.vi"("section"=w21, "default value"=30, "key"="FrameRate", "refnum"=w6) -> ("value"=w16:i32, "refnum out"=w5:T21)  [unwired: 1 in, 5 out]
  n142 = control-ref of="Tree"() -> (w2:refnum<vi>)
  n143 = property on="Listbox" class="LstBox (strict)"("Item Symbols"=i32[] [], "Item Names"=w28) -> ()  [unwired: 2 in, 2 out]
  n144 = Close File(refnum=w7) -> ()  [unwired: 1 in, 2 out]
  n145 = call-poly <vilib>:"Read Key.vi"("section"=w21, "default value"=30, "key"="Compression", "refnum"=w5) -> ("value"=w15:i32, "refnum out"=w3:T21)  [unwired: 1 in, 5 out]
  n146 = while {
    tunnel: [w266] -> _
    tunnel: w2 -> [w265]
    i -> [w266]
    stop <- FALSE stop-if-true
    n147 = Wait (ms)(milliseconds to wait=u32 60) -> ()  [unwired: 1 out]
    n148 = case shown="\"Variables\"" "Viewer" {
      tunnel: w265 -> [_ w270]
      frame Default {
      }
      frame "Variables" {
        n149 = call <vilib>:"NT Read and Format Entries as Tree.vi"("Tree Refnum"=w270) -> ()  [unwired: 9 in, 2 out]
      }
    }
  }
  n150 = control-ref of="Test Tree"() -> (w1:refnum<vi>)
  n151 = while {
    tunnel: w13 -> [w275]
    shift-right: [w274] -> _
    shift-left: w3 -> [w273]
    tunnel: [w272] -> _
    tunnel: w1 -> [w271]
    i -> [w272]
    stop <- FALSE stop-if-true
    (unwired) 0.0 ("Meter")
    n152 = event shown="[0] Timeout" {
      selector: _ -> [_ _ _ _ _ _ _ _ _ _ _ _ _]
      dyn-events: _ -> [_ _ _ _ _ _ _ _ _ _ _ _ _]
      timeout: u32 60 ("milliseconds to wait") -> [_ _ _ _ _ _ _ _ _ _ _ _ _]
      tunnel: w271 -> [w285 _ _ _ _ _ _ _ _ _ _ _ _]
      tunnel: "Test Tree" -> [_ _ _ _ _ _ _ _ w479 w487 w489 w493 w501]
      tunnel: w275 -> [_ w307 _ _ _ _ w443 w473 _ _ _ _ _]
      tunnel: [w279 w306 _ w409 w417 w429 w442 w466 w478 w485 w488 w492 w500] -> w274
      tunnel: w273 -> [w279 w306 _ w409 w417 w429 w441 w466 w478 w485 w488 w492 w500]
      event Timeout {
        w284 = enum16{"Update", "Clear"}[] [enum."Clear", enum."Clear", enum."Clear", enum."Clear", enum."Update", enum."Update", enum."Clear"] items=["Update", "Clear"]
        n153 = event-data() -> ()  [unwired: 1 in, 1 out]
        n154 = local read "Mode"() -> (w282:T2)
        n155 = Index Array(array=w284, index=w282) -> (element=w283:enum16{"Update", "Clear"})
        n156 = call <vilib>:"NT Read String.vi"("Name"="TestMode/TestName") -> ("String"=w288:string)  [unwired: 9 in, 1 out]
        n157 = case shown="\"Ops\", Default" "Dashboard Tab" {
          tunnel: w285 -> [_ w298]
          tunnel: "/TestMode/Automatic/" ("Name Pattern") -> [_ w297]
          tunnel: w283 -> [_ w296]
          tunnel: w282 -> [_ w294]
          frame "Ops", Default {
          }
          frame "Test" {
            w293 = -2 ("Active Item:Row Number")
            n158 = call <vilib>:"NT Read and Format Entries as Tree.vi"("Operation"=w296, "Name Pattern"=w297, "Tree Refnum"=w298) -> ()  [unwired: 7 in, 2 out]
            n159 = Index Array(array=u32[] [14013909, 14013909, 14013909, 14013909, 14013909, 16777215, 14013909], index=w294) -> (element=w292:u32)
            n160 = property on="Test Tree" class="Tree (strict)"("Active Item Row Number"=w293, "ActiveColNum"=w293, "CellBG"=w292, "Active Item Row Number"=-1 ("Active Item:Row Number"), "CellBG"=u32 5789784 ("Color Box")) -> ()  [unwired: 2 in, 2 out]
          }
        }
        n161 = case shown="\"\"" w288 {
          tunnel: "TestMode/TestProgress" ("Name") -> [w300 _]
          tunnel: "TestMode/TestProgressText" ("Name") -> [w299 _]
          frame Default {
            n162 = call <vilib>:"NT Read Number.vi"("Name"=w300) -> ("Numeric"=w301:dbl)  [unwired: 9 in, 1 out]
            n163 = call <vilib>:"NT Read String.vi"("Name"=w299) -> ("String"=w302:string)  [unwired: 9 in, 1 out]
            n164 = Bundle("Numeric"=w301, "String"=w302) -> (→"Progress":cluster{"Numeric":dbl, "String":string})  [unwired: 1 in]
          }
          frame "" {
            n165 = property on="Progress" class="Clust (strict)"("Visible"=FALSE) -> ()  [unwired: 2 in, 2 out]
            n166 = local write "Test Name"(u16 0) -> ()
          }
        }
      }
      event "Test Tree": Value Change {
        # "Show appropriate\ncontrols"
        n167 = event-data() -> ("CtlRef"=w310:refnum<vi>, "NewVal"=w308:string)  [unwired: 1 in]
        n168 = call <vilib>:"WPI_UtilitiesGetTreeIOName.vi"("NewVal"=w308, "TreeControl in"=w310) -> ("I/O Name"=w311:string)  [unwired: 9 in]
        n169 = case shown="\"Camera\"" w311 {
          selector: w311 -> [_ w318 _ w336 w345 _]
          tunnel: w308 -> [_ _ w333 w335 _ w352]
          tunnel: w307 -> [_ _ _ _ _ w351]
          frame Default {
            w313 = FALSE ("Visible")
            w312 = FALSE ("Visible")
            n170 = property on="Motor" class="Clust (strict)"("Visible"=w312) -> ()  [unwired: 2 in, 2 out]
            n171 = property on="Ring" class="Ring (strict)"("Visible"=w312) -> ()  [unwired: 2 in, 2 out]
            n172 = property on="Rev/Fwd" class="Clust (strict)"("Visible"=w313) -> ()  [unwired: 2 in, 2 out]
            n173 = property on="On/Off" class="Bool (strict)"("Visible"=w313) -> ()  [unwired: 2 in, 2 out]
            n174 = property on="Slider" class="Slide (strict)"("Visible"=w313) -> ()  [unwired: 2 in, 2 out]
          }
          frame "Motor", "PWM" {
            w319 = FALSE ("Visible")
            n175 = case shown="\"Motor\", Default" w318 {
              tunnel: [1.0 ("Value") -1.0 ("Value")] -> w317
              tunnel: [255.0 ("Value") 1.0 ("Value")] -> w316
              tunnel: [128.0 ("Value") 0.0 ("Value")] -> w315
              tunnel: [64.0 ("Value") 0.5 ("Value")] -> w314
              frame "PWM" {
              }
              frame "Motor", Default {
              }
            }
            n176 = property on="Motor" class="Clust (strict)"("Visible"=TRUE) -> ()  [unwired: 2 in, 2 out]
            n177 = property on="Value" class="Slide (strict)"("Value"=w315, "Scale.Minimum"=w317, "Scale.Maximum"=w316, "Scale.Increment"=w314) -> ()  [unwired: 2 in, 2 out]
            n178 = property on="On/Off" class="Bool (strict)"("Visible"=w319) -> ()  [unwired: 2 in, 2 out]
            n179 = property on="Slider" class="Slide (strict)"("Visible"=w319) -> ()  [unwired: 2 in, 2 out]
            n180 = property on="Ring" class="Ring (strict)"("Visible"=w319) -> ()  [unwired: 2 in, 2 out]
            n181 = property on="Rev/Fwd" class="Clust (strict)"("Visible"=w319) -> ()  [unwired: 2 in, 2 out]
          }
          frame "Servo" {
            w331 = FALSE ("Visible")
            n182 = call <vilib>:"NT Read Number.vi"("Name"=w333) -> ("Numeric"=w332:dbl)  [unwired: 9 in, 1 out]
            n183 = property on="Slider" class="Slide (strict)"("Visible"=TRUE, "Scale.Maximum"=170.0 ("Scale.Range:Maximum")) -> ()  [unwired: 2 in, 2 out]
            n184 = local write "Slider"(w332) -> ()
            n185 = property on="Motor" class="Clust (strict)"("Visible"=w331) -> ()  [unwired: 2 in, 2 out]
            n186 = property on="Rev/Fwd" class="Clust (strict)"("Visible"=w331) -> ()  [unwired: 2 in, 2 out]
            n187 = property on="On/Off" class="Bool (strict)"("Visible"=w331) -> ()  [unwired: 2 in, 2 out]
            n188 = property on="Ring" class="Ring (strict)"("Visible"=w331) -> ()  [unwired: 2 in, 2 out]
          }
          frame "Relay", "Solenoid" {
            w334 = FALSE ("Visible")
            n189 = property on="Motor" class="Clust (strict)"("Visible"=w334) -> ()  [unwired: 2 in, 2 out]
            n190 = property on="Slider" class="Slide (strict)"("Visible"=w334) -> ()  [unwired: 2 in, 2 out]
            n191 = Search and Replace String(input string=w335, search string="/Value  **", replace string="/Direction") -> (result string=w341:string)  [unwired: 5 in, 3 out]
            n192 = property on="Ring" class="Ring (strict)"("Visible"=w334) -> ()  [unwired: 2 in, 2 out]
            n193 = call <vilib>:"NT Read String.vi"("Name"=w341) -> ("String"=w339:string)  [unwired: 9 in, 1 out]
            n194 = Equal?(x="Both directions", y=w339) -> (x = y?=w337:bool)
            n195 = Not(x=w337) -> (.not. x?=w338:bool)
            n196 = property on="Rev/Fwd" class="Clust (strict)"("Visible"=w337) -> ()  [unwired: 2 in, 2 out]
            n197 = property on="On/Off" class="Bool (strict)"("Visible"=w338, "Caption.Text"=w336) -> ()  [unwired: 2 in, 2 out]
          }
          frame "Compressor", "Digital Out" {
            w344 = FALSE ("Visible")
            # "Get direction and finish"
            n198 = property on="Motor" class="Clust (strict)"("Visible"=w344) -> ()  [unwired: 2 in, 2 out]
            n199 = property on="Slider" class="Slide (strict)"("Visible"=w344) -> ()  [unwired: 2 in, 2 out]
            n200 = property on="Ring" class="Ring (strict)"("Visible"=w344) -> ()  [unwired: 2 in, 2 out]
            n201 = property on="On/Off" class="Bool (strict)"("Visible"=TRUE, "Caption.Text"=w345) -> ()  [unwired: 2 in, 2 out]
            n202 = property on="Rev/Fwd" class="Clust (strict)"("Visible"=FALSE) -> ()  [unwired: 2 in, 2 out]
          }
          frame "Camera" {
            n203 = call <vilib>:"Get Last Path Segment.vi"("String in"=w352) -> ("String out"=w353:string)  [unwired: 10 in]
            n204 = property on="On/Off" class="Bool (strict)"("Visible"=FALSE) -> ()  [unwired: 2 in, 2 out]
            n205 = property on="Motor" class="Clust (strict)"("Visible"=FALSE) -> ()  [unwired: 2 in, 2 out]
            n206 = property on="Rev/Fwd" class="Clust (strict)"("Visible"=FALSE) -> ()  [unwired: 2 in, 2 out]
            n207 = case shown="\"White Balance  **\"" w353 {
              tunnel: w352 -> [w359 w368 w377 w386 w395 _ w401]
              tunnel: w351 -> [w357 w365 w374 w383 w392 _ _]
              frame "Size  **" {
                n208 = Index Array(array=w357) -> (element=w356:cluster{string[]})  [unwired: 1 in]
                n209 = call <vilib>:"NT Read String.vi"("Name"=w359) -> ("String"=w358:string)  [unwired: 9 in, 1 out]
                n210 = Unbundle(w356) -> (w354:string[])
                n211 = Match First String(2:w354, 3:w358) -> (0:w355:i32)  [unwired: 1 out]
                n212 = property on="Ring" class="Ring (strict)"("Value"=w355, "Strings []"=w354) -> ()  [unwired: 2 in, 2 out]
                n213 = property on="Ring" class="Ring (strict)"("Visible"=TRUE) -> ()  [unwired: 2 in, 2 out]
                n214 = property on="Slider" class="Slide (strict)"("Visible"=FALSE) -> ()  [unwired: 2 in, 2 out]
              }
              frame "White Balance  **" {
                n215 = Index Array(array=w365, index=1) -> (element=w366:cluster{string[]})
                n216 = call <vilib>:"NT Read String.vi"("Name"=w368) -> ("String"=w367:string)  [unwired: 9 in, 1 out]
                n217 = Unbundle(w366) -> (w363:string[])
                n218 = Match First String(2:w363, 3:w367) -> (0:w362:i32)  [unwired: 1 out]
                n219 = property on="Ring" class="Ring (strict)"("Value"=w362, "Strings []"=w363) -> ()  [unwired: 2 in, 2 out]
                n220 = property on="Ring" class="Ring (strict)"("Visible"=TRUE) -> ()  [unwired: 2 in, 2 out]
                n221 = property on="Slider" class="Slide (strict)"("Visible"=FALSE) -> ()  [unwired: 2 in, 2 out]
              }
              frame "Exposure  **" {
                n222 = Index Array(array=w374, index=2) -> (element=w375:cluster{string[]})
                n223 = call <vilib>:"NT Read String.vi"("Name"=w377) -> ("String"=w376:string)  [unwired: 9 in, 1 out]
                n224 = Unbundle(w375) -> (w371:string[])
                n225 = Match First String(2:w371, 3:w376) -> (0:w372:i32)  [unwired: 1 out]
                n226 = property on="Ring" class="Ring (strict)"("Value"=w372, "Strings []"=w371) -> ()  [unwired: 2 in, 2 out]
                n227 = property on="Ring" class="Ring (strict)"("Visible"=TRUE) -> ()  [unwired: 2 in, 2 out]
                n228 = property on="Slider" class="Slide (strict)"("Visible"=FALSE) -> ()  [unwired: 2 in, 2 out]
              }
              frame "Exposure Priority  **" {
                n229 = Index Array(array=w383, index=3) -> (element=w384:cluster{string[]})
                n230 = call <vilib>:"NT Read String.vi"("Name"=w386) -> ("String"=w385:string)  [unwired: 9 in, 1 out]
                n231 = Unbundle(w384) -> (w380:string[])
                n232 = Match First String(2:w380, 3:w385) -> (0:w381:i32)  [unwired: 1 out]
                n233 = property on="Ring" class="Ring (strict)"("Value"=w381, "Strings []"=w380) -> ()  [unwired: 2 in, 2 out]
                n234 = property on="Ring" class="Ring (strict)"("Visible"=TRUE) -> ()  [unwired: 2 in, 2 out]
                n235 = property on="Slider" class="Slide (strict)"("Visible"=FALSE) -> ()  [unwired: 2 in, 2 out]
              }
              frame "Color Enable  **" {
                n236 = Index Array(array=w392, index=4) -> (element=w393:cluster{string[]})
                n237 = call <vilib>:"NT Read String.vi"("Name"=w395) -> ("String"=w394:string)  [unwired: 9 in, 1 out]
                n238 = Unbundle(w393) -> (w389:string[])
                n239 = Match First String(2:w389, 3:w394) -> (0:w390:i32)  [unwired: 1 out]
                n240 = property on="Ring" class="Ring (strict)"("Value"=w390, "Strings []"=w389) -> ()  [unwired: 2 in, 2 out]
                n241 = property on="Ring" class="Ring (strict)"("Visible"=TRUE) -> ()  [unwired: 2 in, 2 out]
                n242 = property on="Slider" class="Slide (strict)"("Visible"=FALSE) -> ()  [unwired: 2 in, 2 out]
              }
              frame Default {
                n243 = property on="Ring" class="Ring (strict)"("Visible"=FALSE) -> ()  [unwired: 2 in, 2 out]
                n244 = property on="Slider" class="Slide (strict)"("Visible"=FALSE) -> ()  [unwired: 2 in, 2 out]
              }
              frame "Brightness  **", "Color Level  **", "Compression  **", "FPS  **", "Sharpness  **" {
                n245 = call <vilib>:"NT Read Number.vi"("Name"=w401) -> ("Numeric"=w400:dbl)  [unwired: 9 in, 1 out]
                n246 = local write "Slider"(w400) -> ()
                n247 = property on="Slider" class="Slide (strict)"("Visible"=TRUE, "Scale.Maximum"=100.0 ("Scale.Range:Maximum")) -> ()  [unwired: 2 in, 2 out]
                n248 = property on="Ring" class="Ring (strict)"("Visible"=FALSE) -> ()  [unwired: 2 in, 2 out]
              }
            }
          }
        }
        n249 = property on="Progress" class="Clust (strict)"("Visible"=FALSE) -> ()  [unwired: 2 in, 2 out]
      }
      event "Test Name": Mouse Enter {
        # "Populate the ring with the list of tests"
        n250 = event-data() -> ()  [unwired: 1 in, 1 out]
        n251 = call <vilib>:"NT Read String Array.vi"("Name"="TestMode/TestList") -> ("String Array"=w408:string[])  [unwired: 9 in, 1 out]
        n252 = Build Array (concatenate)("Select the test to run...", w408) -> (w407:string[])
        n253 = property on="Test Name" class="Ring (strict)"("Strings []"=w407) -> ()  [unwired: 2 in, 2 out]
      }
      event "Test Name": Value Change {
        w410 = FALSE ("Visible")
        # "Tell the robot the test name to run"
        n254 = event-data() -> ("NewVal"=w414:u16)  [unwired: 1 in]
        n255 = property on="Test Name" class="Ring (strict)"() -> ("Strings []"=w415:string[])  [unwired: 2 in, 2 out]
        n256 = local write "Progress"(T8 {"Test Progress"=0, "Test Progress Text"=""} ("Progress")) -> ()
        n257 = Index Array(array=w415, index=w414) -> (element=w413:string)
        n258 = call <vilib>:"NT Write String.vi"("String"=w413, "Name"="TestMode/TestName") -> ()  [unwired: 9 in, 1 out]
        n259 = property on="Progress" class="Clust (strict)"("Visible"=TRUE) -> ()  [unwired: 2 in, 2 out]
        n260 = property on="Motor" class="Clust (strict)"("Visible"=w410) -> ()  [unwired: 2 in, 2 out]
        n261 = property on="Slider" class="Slide (strict)"("Visible"=w410) -> ()  [unwired: 2 in, 2 out]
        n262 = property on="On/Off" class="Bool (strict)"("Visible"=w410) -> ()  [unwired: 2 in, 2 out]
        n263 = property on="Rev/Fwd" class="Clust (strict)"("Visible"=w410) -> ()  [unwired: 2 in, 2 out]
        n264 = property on="Ring" class="Ring (strict)"("Visible"=w410) -> ()  [unwired: 2 in, 2 out]
      }
      event "Listbox": Double Click {
        n265 = event-data() -> ("PlatMods.Shift"=w418:bool, "Row"=w420:i32)  [unwired: 1 in]
        n266 = case shown="False" w418 {
          tunnel: w420 -> [w424 _]
          tunnel: 1 -> [w423 _]
          frame False {
            n267 = property on="Listbox" class="LstBox (strict)"() -> ("Item Symbols"=w422:i32[])  [unwired: 2 in, 2 out]
            n268 = Replace Array Subset(array=w422, new element=w423, index=w424) -> (w421:i32[])
            n269 = property on="Listbox" class="LstBox (strict)"("Item Symbols"=w421) -> ()  [unwired: 2 in, 2 out]
          }
          frame True {
            w425 = 0 ("Top Row")
            n270 = property on="Listbox" class="LstBox (strict)"() -> ("Number of Rows"=w427:u32)  [unwired: 2 in, 2 out]
            n271 = Initialize Array(0, w427) -> (w426:i32[])
            n272 = property on="Listbox" class="LstBox (strict)"("Top Row"=w425, "Value"=w425, "Item Symbols"=w426) -> ()  [unwired: 2 in, 2 out]
          }
        }
      }
      event "Listbox": Key Down {
        n273 = event-data() -> ("VKey"=w431:T22)  [unwired: 1 in]
        n274 = case shown="\"Left\", \"Right\"" w431 {
          selector: w431 -> [w436 _]
          tunnel: eventvkey."Left" ("VKey") -> [w434 _]
          frame "Left", "Right" {
            n275 = Equal?(x=w434, y=w436) -> (x = y?=w435:bool)
            n276 = Select(t=0, s=w435, f=1) -> (s? t:f=w437:i32)
            n277 = property on="Listbox" class="LstBox (strict)"() -> ("Item Symbols"=w440:i32[])  [unwired: 2 in, 2 out]
            n278 = Replace Array Subset(array=w440, new element=w437, index="Listbox") -> (w439:i32[])
            n279 = property on="Listbox" class="LstBox (strict)"("Item Symbols"=w439) -> ()  [unwired: 2 in, 2 out]
          }
          frame Default {
          }
        }
      }
      event "DB Camera Config": Value Change {
        n280 = event-data() -> ("NewVal"=w444:bool)  [unwired: 1 in]
        n281 = case shown="False" w444 {
          tunnel: w443 -> [w453 _]
          tunnel: [w446 w464] -> w442
          tunnel: w441 -> [w445 w464]
          frame False {
            w460 = "Camera"
            w463 = FALSE ("Visible")
            n282 = local read "Camera Settings"() -> (w452:T1)
            n283 = Index Array(array=w453) -> (element=w456:cluster{string[]})  [unwired: 1 in]
            n284 = Unbundle(w452) -> ("Frate Rate"=w451:i32, "Compression"=w450:i32, "Size"=w454:u16)
            n285 = Unbundle(w456) -> (w455:string[])
            n286 = Index Array(array=w455, index=w454) -> (element=w449:string)
            n287 = call-poly <vilib>:"Write Key.vi"("section"=w460, "value"=w449, "key"="Size", "refnum"=w445) -> ("refnum out"=w462:T21)  [unwired: 2 in, 5 out]
            n288 = call-poly <vilib>:"Write Key.vi"("section"=w460, "value"=w451, "key"="FrameRate", "refnum"=w462) -> ("refnum out"=w461:T21)  [unwired: 1 in, 6 out]
            n289 = property on="Camera Settings" class="Clust (strict)"("Visible"=w463) -> ()  [unwired: 2 in, 2 out]
            n290 = local write "DB Camera Config"(w463) -> ()
            n291 = call-poly <vilib>:"Write Key.vi"("section"=w460, "value"=w450, "key"="Compression", "refnum"=w461) -> ("refnum out"=w447:T21)  [unwired: 1 in, 6 out]
            n292 = call <vilib>:"Close Config Data.vi"("refnum"=w447) -> ("file path"=w448:path)  [unwired: 2 in, 8 out]
            n293 = call <vilib>:"Open Config Data.vi"("configuration file path"=w448) -> ("refnum"=w446:T21)  [unwired: 8 in, 2 out]
          }
          frame True {
            n294 = property on="Camera Settings" class="Clust (strict)"("Visible"=TRUE) -> ()  [unwired: 2 in, 2 out]
          }
        }
      }
      event "Camera Settings": Value Change {
        n295 = event-data() -> ("NewVal"=w477:T1)  [unwired: 1 in]
        n296 = Index Array(array=w473) -> (element=w472:cluster{string[]})  [unwired: 1 in]
        n297 = Unbundle(w477) -> ("Frate Rate"=w468:i32, "Compression"=w467:i32, "Size"=w470:u16)
        n298 = Unbundle(w472) -> (w471:string[])
        n299 = Index Array(array=w471, index=w470) -> (element=w469:string)
        n300 = Format Into String(format string="%s   %dfps   %d%%", w469, w468, w467) -> (resulting string=w474:string)  [unwired: 2 in, 1 out]
        n301 = Build Array(w474) -> (w475:string[])
        n302 = property on="DB Camera Config" class="Bool (strict)"("Strings [4]"=w475) -> ()  [unwired: 2 in, 2 out]
      }
      event "Motor.Enable": Value Change {
        n303 = event-data() -> ("NewVal"=w483:bool)  [unwired: 1 in]
        n304 = Unbundle("Motor") -> ("Value"=w482:dbl)  [unwired: 1 out]
        n305 = Select(t=w482, s=w483, f=0.0) -> (s? t:f=w480:dbl)
        n306 = call <vilib>:"NT Write Number.vi"("Numeric"=w480, "Name"=w479) -> ()  [unwired: 9 in, 1 out]
      }
      event "Slider": Value Change {
        n307 = event-data() -> ("NewVal"=w486:dbl)  [unwired: 1 in]
        n308 = call <vilib>:"NT Write Number.vi"("Numeric"=w486, "Name"=w487) -> ()  [unwired: 9 in, 1 out]
      }
      event "On/Off": Value Change {
        n309 = event-data() -> ("NewVal"=w491:bool)  [unwired: 1 in]
        n310 = Boolean To (0,1)(Boolean=w491) -> (0, 1=w490:i16)
        n311 = call <vilib>:"NT Write Number.vi"("Numeric"=w490, "Name"=w489) -> ()  [unwired: 9 in, 1 out]
      }
      event "Rev/Fwd": Value Change {
        n312 = event-data() -> ("NewVal.Forward"=w499:bool, "NewVal.Reverse"=w498:bool)  [unwired: 1 in]
        n313 = Boolean To (0,1)(Boolean=w499) -> (0, 1=w495:i16)
        n314 = Boolean To (0,1)(Boolean=w498) -> (0, 1=w497:i16)
        n315 = Negate(x=w497) -> (-x=w496:i16)
        n316 = Add(x=w495, y=w496) -> (x+y=w494:i16)
        n317 = call <vilib>:"NT Write Number.vi"("Numeric"=w494, "Name"=w493) -> ()  [unwired: 9 in, 1 out]
      }
      event "Ring": Value Change {
        n318 = event-data() -> ("NewVal"=w503:u16)  [unwired: 1 in]
        n319 = property on="Ring" class="Ring (strict)"() -> ("Strings []"=w504:string[])  [unwired: 2 in, 2 out]
        n320 = Index Array(array=w504, index=w503) -> (element=w502:string)
        n321 = call <vilib>:"NT Write String.vi"("String"=w502, "Name"=w501) -> ()  [unwired: 9 in, 1 out]
      }
    }
  }
  n322 = Index Array(array=w13) -> (element=w14:cluster{string[]})  [unwired: 1 in]
  n323 = Unbundle(w14) -> (w12:string[])
  n324 = Match First String(2:w12, 3:w11) -> (0:w10:i32)  [unwired: 1 out]
  n325 = Bundle("value"=w16, "value"=w15, "index"=w10) -> (w4:cluster{"value":i32, "value":i32, "index":i32})  [unwired: 1 out]
  n326 = property on="On/Off" class="Bool (strict)"("Visible"=w27) -> ()  [unwired: 2 in, 2 out]
  n327 = property on="Motor" class="Clust (strict)"("Visible"=w27) -> ()  [unwired: 2 in, 2 out]
  n328 = property on="Progress" class="Clust (strict)"("Visible"=w27) -> ()  [unwired: 2 in, 2 out]
  n329 = property on="Ring" class="Ring (strict)"("Visible"=w27) -> ()  [unwired: 2 in, 2 out]
  n330 = property on="Camera Settings" class="Clust (strict)"("Val(Sgnl)"=w4) -> ()  [unwired: 2 in, 2 out]
  n331 = property on="Rev/Fwd" class="Clust (strict)"("Visible"=w27) -> ()  [unwired: 2 in, 2 out]
  n332 = property on="Camera Settings" class="Clust (strict)"("Visible"=w27) -> ()  [unwired: 2 in, 2 out]
  n333 = local write "DB Camera Config"(w27) -> ()
